vi "write_cluster_params.vi"(8 "error in (no error)":errorcluster, 10 "cluster":variant, 11 "variant in":variant) -> (0 "error out":errorcluster, 3 "variant out":variant)   [LabVIEW 2015]
uses:
  <vilib>/Utility/Data Type/Type Definitions/Data Type.ctl
  <vilib>/Utility/Data Type/NI_Data Type.lvlib
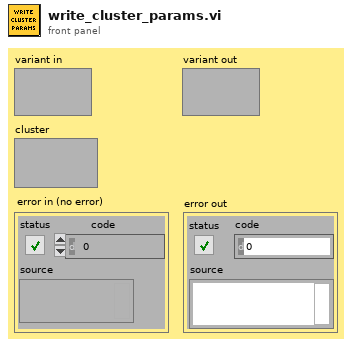
[diagram p1: front panel]
types:
  T1 = typedef "NI_Data Type.lvlib/Data Type.ctl" = enum8{"Invalid Type", "Void", "I8", "I16", "I32", "I64", "U8", "U16", "U32", "U64", "Single Float", "Double Float", "Extended Float", "Single Complex", "Double Complex", "Extended Complex", "Enum U8", "Enum U16", "Enum U32", "Enum U64", "Single Float With Unit", "Double Float With Unit", "Extended Float With Unit", "Single Complex with Unit", "Double Complex with Unit", "Extended Complex with Unit", "Boolean", "String", "Path", "Picture", "Tag", "Array", "Cluster", "Variant", "LV Variant", "Waveform", "Timestamp", "Digital Waveform", "Digital Data", "ExpressData", "Refnum", "External Data", "VI", "Poly VI", "LabVIEW Class Instance", "Fixed Point"}
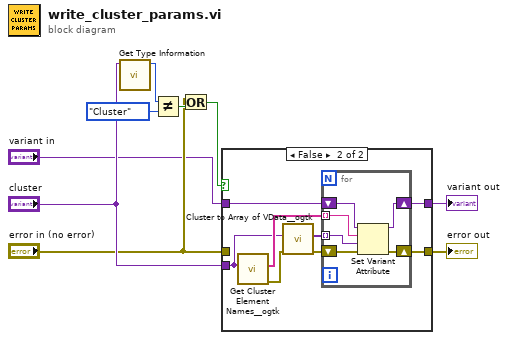
[diagram p0: block diagram]
diagram:
  n1 = call <vilib>:"Get Type Information.vi"("Variant"="cluster") -> ("Type"=w8:T1)  [unwired: 6 in, 4 out]
  n2 = Not Equal?(x=w8, y=Data_Type."Cluster" ("Type")) -> (x != y?=w6:bool)
  n3 = Or(x="error in (no error)", y=w6) -> (x .or. y?=w5:bool)
  n4 = case shown="False" w5 {
    tunnel: "cluster" -> [_ w16]
    tunnel: [w11 w14] -> w4
    tunnel: "error in (no error)" -> [w11 _]
    tunnel: "variant in" -> [w10 w13]
    tunnel: [w10 w12] -> w1
    frame True {
    }
    frame False {
      n5 = call <userlib>:"Get Cluster Element Names__ogtk.vi"("Cluster"=w16) -> ("error out"=w19:errorcluster, "Element Names"=w17:string[])  [unwired: 9 in]
      n6 = call <userlib>:"Cluster to Array of VData__ogtk.vi"("error in (no error)"=w19, "Cluster"=w16) -> ("error out"=w15:errorcluster, "Array of VData"=w18:variant[])  [unwired: 8 in]
      n7 = for {
        tunnel: w18 -> [w24] mode=indexing
        tunnel: w17 -> [w25] mode=indexing
        shift-right: [w21] -> w14
        shift-left: w15 -> [w20]
        shift-right: [w22] -> w12
        shift-left: w13 -> [w23]
        n8 = Set Variant Attribute(Variant=w23, name=w25, value=w24, error in=w20) -> (Variant out=w22:variant, error out=w21:errorcluster)  [unwired: 1 out]
      }
    }
  }
  "error out" <- w4
  "variant out" <- w1
